vi "Format Fit Output.vi"(5 "Fit Model":T4, 7 "f(x,a)":T1, 8 "Error In":errorcluster, 9 "Fit Results":T2, 10 "Additional Data":variant, 11 "Data in":T3) -> (0 "Error Out":errorcluster, 1 "Fit Parameters Uncertainties Cluster":variant, 3 "Fit Parameters Cluster":variant)   [LabVIEW 2019]
uses:
  Fit Models.ctl
  <vilib>/gmath/NumericalOptimization/LM model function reference.ctl
  <vilib>/Utility/error.llb/DialogType.ctl
  Gaussian Fit Results v2.ctl
  Asymmetric Gaussian Fit Results v2.ctl
  Lorentzian Fit Results v2.ctl
  Asymmetric Lorentzian Fit Results v2.ctl
  Gaussian-Lorentzian Fit Results v2.ctl
  Lorentzian-Gaussian Fit Results v2.ctl
  D-Only Fixed Parameters.ctl
  Two H-Connected Gaussians Fit Parameters.ctl
  Two T-Connected Gaussians Fit Parameters.ctl
  Two H-Connected Asymmetric Gaussians Fit Parameters.ctl
  Two T-Connected Asymmetric Gaussians Fit Parameters.ctl
  Single Exponential Fit Parameters v2.ctl
  Double Exponential Fit Parameters v2.ctl
  2D Gaussian ACF Fit Results.ctl
  2D Gaussian + Blinking ACF Fit Results.ctl
  2D Gaussian + Flow ACF Fit Results.ctl
  3D Gaussian ACF Fit Results.ctl
  3D Gaussian + Blinking ACF Fit Results.ctl
  2D Gaussian ACF & 2D Gaussian ACF + Flow Fit Results.ctl
  <vilib>/Analysis/NI_AALPro.lvlib
  <vilib>/gmath/NI_Gmath.lvlib
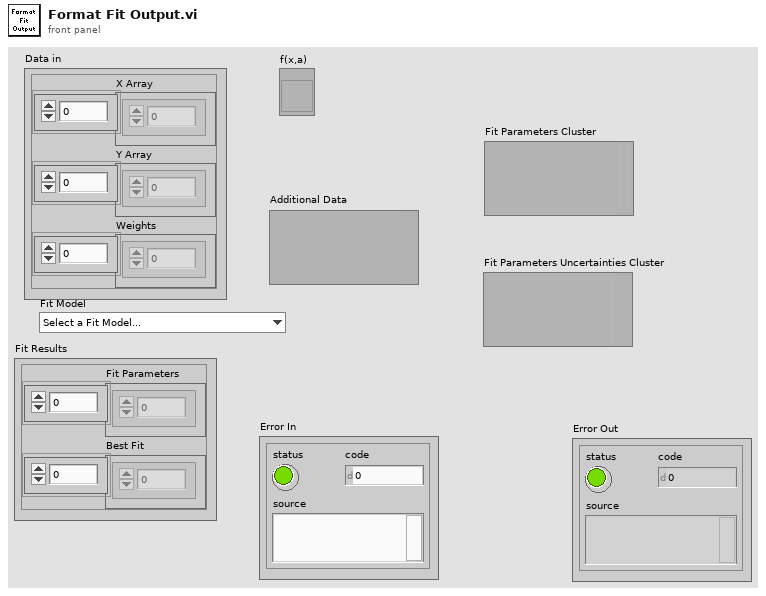
[diagram p1: front panel]
types:
  T1 = typedef "NI_Gmath.lvlib/LM model function reference.ctl" = refnum<vi>
  T2 = cluster{"Fit Parameters":dbl[], "Best Fit":dbl[]}
  T3 = cluster{"X Array":dbl[], "Y Array":dbl[], "Weights":dbl[]}
  T4 = typedef "Fit Models.ctl" = enum16{"Select a Fit Model...", "           Single Peak", "Gaussian", "Asymmetric Gaussian", "Lorentzian", "Asymmetric Lorentzian", "Gaussian/Lorentzian", "Lorentzian/Gaussian", "           Double Peak", "Two Gaussians", "Two Asymmetric Gaussians", "Two H-Connected Gaussians", "Two T-Connected Gaussians", "Two H-Connected Asymmetric Gaussians", "Two T-Connected Asymmetric Gaussians", "           Triple Peak", "Three Gaussians", "Three Asymmetric Gaussians", "              Decays", "Single Exponential", "Two Exponentials", "               ACF", "2D Gaussian ACF", "2D Gaussian + Blinking ACF", "2D Gaussian + Flow ACF", "3D Gaussian ACF", "3D Gaussian + Blinking ACF", "             Multiplot", "2D Gaussian ACF & 2D Gaussian + Flow ACF"}
  T5 = typedef "D-Only Fixed Parameters.ctl" = cluster{"Fix D-only Peak Location":bool, "Peak Location":dbl, "Fix D-only Peak FWHM":bool, "Peak FWHM":dbl}
  T6 = typedef "DialogType.ctl" = u16
  T7 = typedef "Gaussian Fit Results v2.ctl" = cluster{"Amplitude":dbl, "Peak":dbl, "SDV":dbl, "FWHM":dbl, "Integral":dbl, "RMSE":dbl, "R^2":dbl}
  T8 = typedef "Asymmetric Gaussian Fit Results v2.ctl" = cluster{"Amplitude":dbl, "Peak":dbl, "SDV-":dbl, "SDV+":dbl, "Mean":dbl, "SDV":dbl, "FWHM":dbl, "Integral":dbl, "RMSE":dbl, "R^2":dbl}
  T9 = typedef "Lorentzian Fit Results v2.ctl" = cluster{"Amplitude":dbl, "Peak":dbl, "FWHM":dbl, "Integral":dbl, "RMSE":dbl, "R^2":dbl}
  T10 = typedef "Asymmetric Lorentzian Fit Results v2.ctl" = cluster{"Amplitude":dbl, "Peak":dbl, "FWHM-":dbl, "FWHM+":dbl, "Integral":dbl, "RMSE":dbl, "R^2":dbl}
  T11 = typedef "Gaussian-Lorentzian Fit Results v2.ctl" = cluster{"Amplitude":dbl, "Peak":dbl, "SDV-":dbl, "FWHM+":dbl, "Mean":dbl, "FWHM":dbl, "Integral":dbl, " RMSE":dbl, "R^2":dbl}
  T12 = typedef "Lorentzian-Gaussian Fit Results v2.ctl" = cluster{"Amplitude":dbl, "Peak":dbl, "FWHM-":dbl, "SDV+":dbl, "Mean":dbl, "FWHM":dbl, "Integral":dbl, "RMSE":dbl, "R^2":dbl}
  T13 = typedef "Two H-Connected Gaussians Fit Parameters.ctl" = cluster{"Gaussian Parameters":T7[], "Bridge Amplitude ":dbl}
  T14 = typedef "Two T-Connected Gaussians Fit Parameters.ctl" = cluster{"Gaussian Parameters":T7[], "Bridge Amplitude ":dbl, "Bridge Slope":dbl}
  T15 = typedef "Two H-Connected Asymmetric Gaussians Fit Parameters.ctl" = cluster{"Asymmetric Gaussian Parameters":T8[], "Bridge Amplitude":dbl}
  T16 = typedef "Two T-Connected Asymmetric Gaussians Fit Parameters.ctl" = cluster{"Asymmetric Gaussian Parameters":T8[], "Bridge Amplitude":dbl, "Bridge Slope":dbl}
  T17 = typedef "Single Exponential Fit Parameters v2.ctl" = cluster{"Amplitude":dbl, "Time Constant":dbl, "Mean":dbl, "SDV":dbl, "FWHM":dbl, "Integral":dbl, "MSE":dbl, "R^2":dbl}
  T18 = typedef "Double Exponential Fit Parameters v2.ctl" = cluster{"A1":dbl, "tau1":dbl, "A2":dbl, "tau2":dbl, "Mean":dbl, "SDV":dbl, "Integral":dbl, "MSE":dbl, "R^2":dbl}
  T19 = typedef "2D Gaussian ACF Fit Results.ctl" = cluster{"Amplitude":dbl, "Diffusion Time":dbl, "RMSE":dbl, "R^2":dbl}
  T20 = typedef "2D Gaussian + Blinking ACF Fit Results.ctl" = cluster{"Amplitude":dbl, "Diffusion Time":dbl, "Blinking Fraction":dbl, "Blinking Time Constant":dbl, "RMSE":dbl, "R^2":dbl}
  T21 = typedef "2D Gaussian + Flow ACF Fit Results.ctl" = cluster{"Amplitude":dbl, "Diffusion Time":dbl, "Translation Time":dbl, "RMSE":dbl, "R^2":dbl}
  T22 = typedef "3D Gaussian ACF Fit Results.ctl" = cluster{"Amplitude":dbl, "Diffusion Time":dbl, "Aspect Ratio":dbl, "RMSE":dbl, "R^2":dbl}
  T23 = typedef "3D Gaussian + Blinking ACF Fit Results.ctl" = cluster{"Amplitude":dbl, "Diffusion Time":dbl, "Aspect Ratio":dbl, "Blinking Fraction":dbl, "Blinking Time Constant":dbl, "RMSE":dbl, "R^2":dbl}
  T24 = typedef "2D Gaussian ACF & 2D Gaussian ACF + Flow Fit Results.ctl" = cluster{"Amplitude 1":dbl, "Diffusion Time":dbl, "Amplitude 2":dbl, "Translation Time":dbl, "RMSE":dbl, "R^2":dbl}
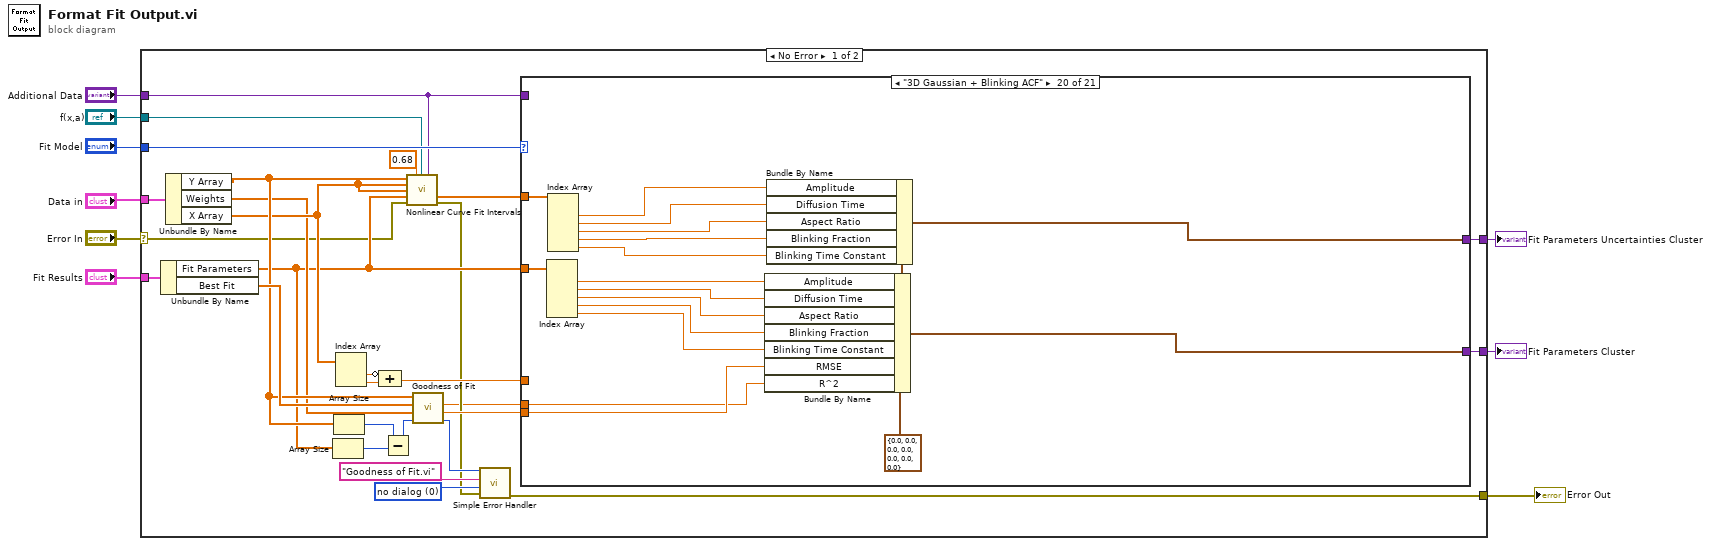
[diagram p0: block diagram]
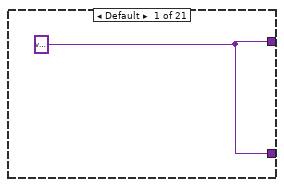
[diagram p2: hidden frame]
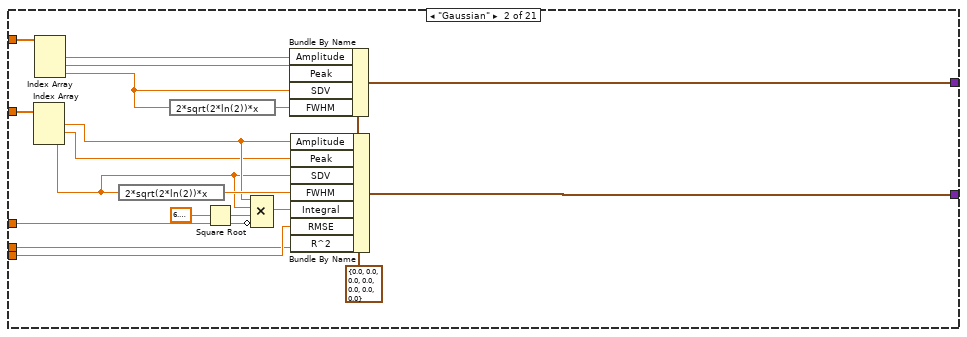
[diagram p3: hidden frame]
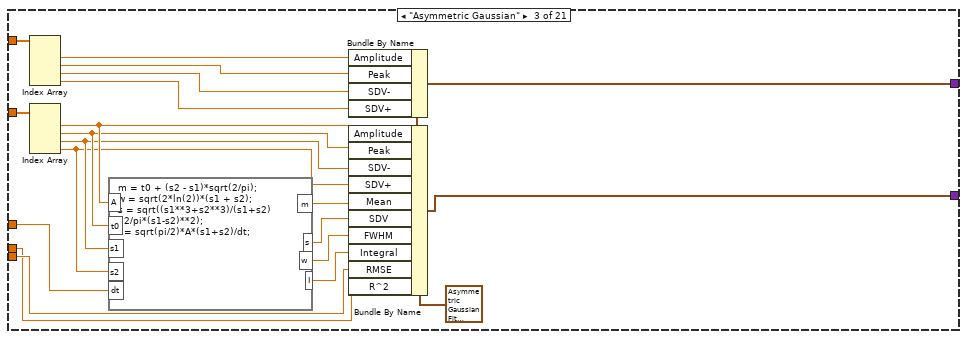
[diagram p4: hidden frame]
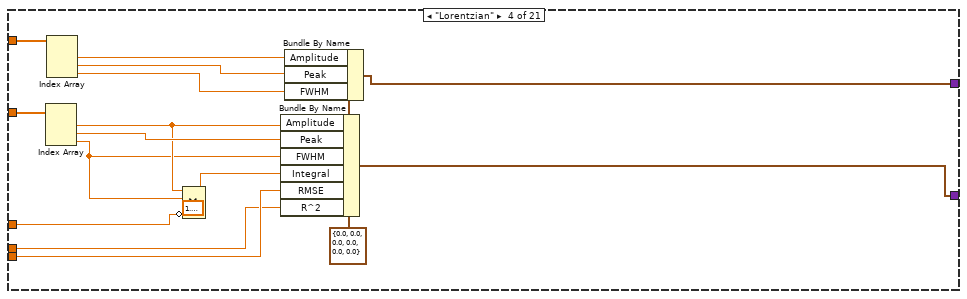
[diagram p5: hidden frame]
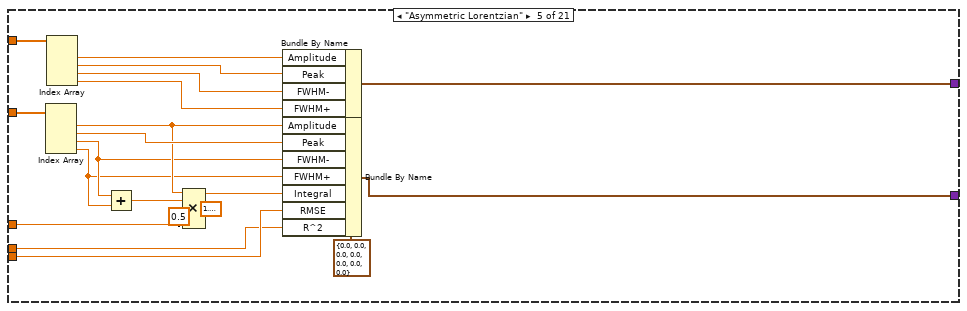
[diagram p6: hidden frame]
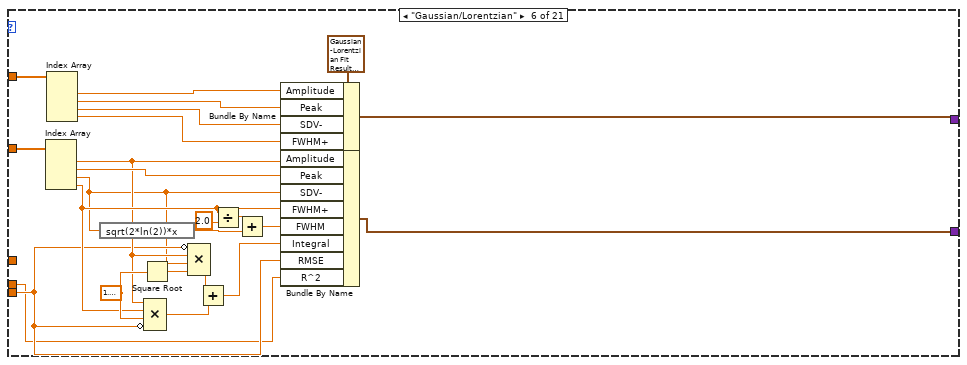
[diagram p7: hidden frame]
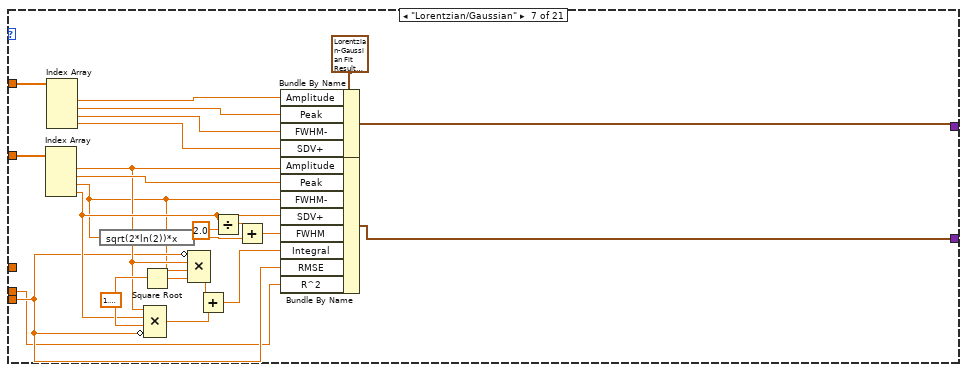
[diagram p8: hidden frame]
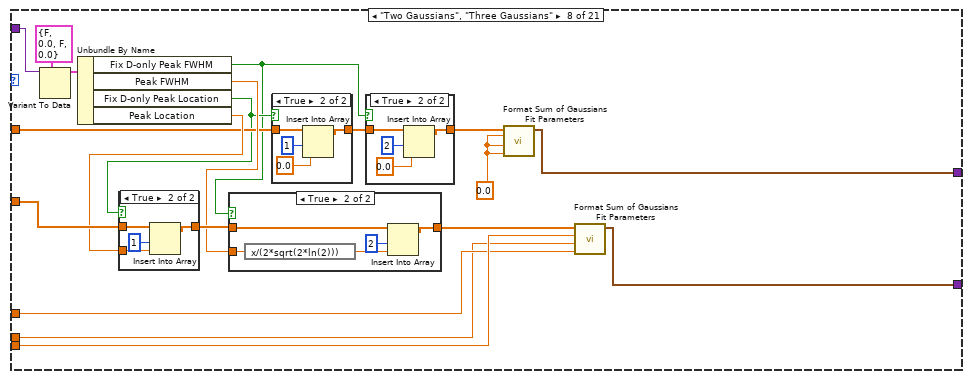
[diagram p9: hidden frame]
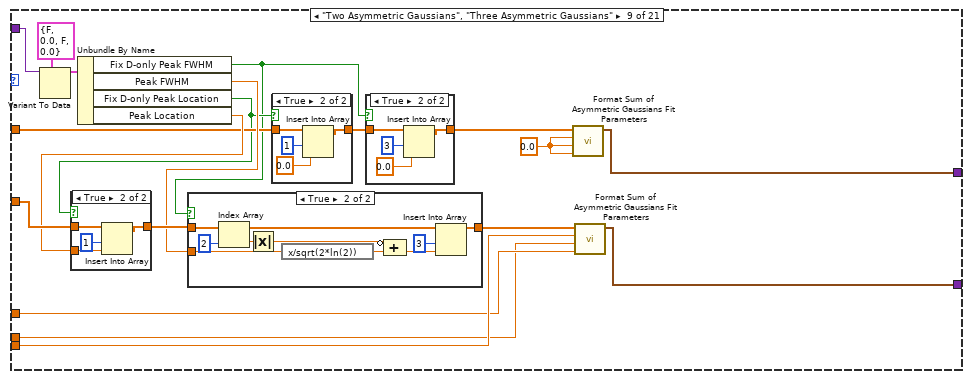
[diagram p14: hidden frame]
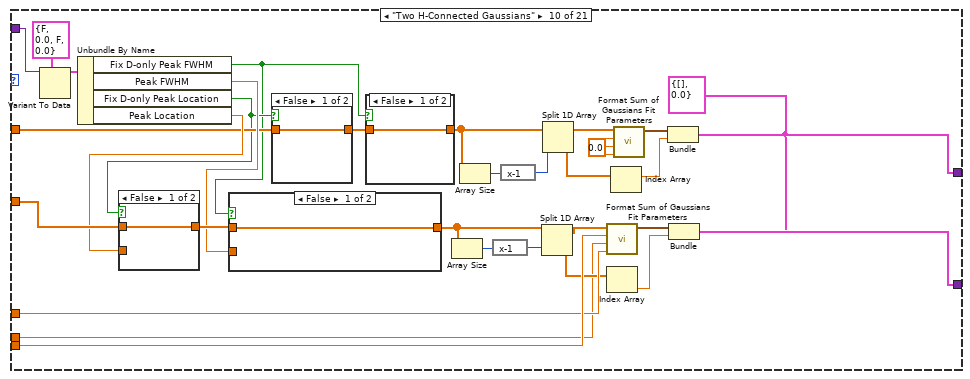
[diagram p19: hidden frame]
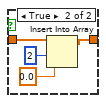
[diagram p20: hidden frame]
diagram:
  n1 = case shown="No Error" "Error In" {
    selector: "Error In" -> [w19 w589]
    tunnel: [w37 _] -> w9
    tunnel: [w36 _] -> w8
    tunnel: "Data in" -> [w28 _]
    tunnel: "Fit Results" -> [w27 _]
    tunnel: "Fit Model" -> [w25 _]
    tunnel: "f(x,a)" -> [w18 _]
    tunnel: [w13 w589] -> w2
    tunnel: "Additional Data" -> [w11 _]
    frame No Error {
      w15 = T6 0 items=["no dialog", "OK message", "continue or stop message", "OK message + warnings", "continue/stop + warnings"] ("type of dialog (OK msg:1)")
      n2 = Unbundle By Name(w27) -> ("Fit Parameters"=w21:dbl[], "Best Fit"=w26:dbl[])
      n3 = Unbundle By Name(w28) -> ("Y Array"=w24:dbl[], "Weights"=w22:dbl[], "X Array"=w23:dbl[])
      n4 = Array Size(array=w21) -> (size(s)=w31:i32)
      n5 = Array Size(array=w24) -> (size(s)=w32:i32)
      n6 = Index Array(array=w23) -> (element #1=w33:dbl, element #2=w35:dbl)  [unwired: 2 in]
      n7 = Compound Arithmetic op=ADD(invert w33, w35) -> (w34:dbl)
      n8 = Subtract(x=w32, y=w31) -> (x-y=w30:i32)
      n9 = call <vilib>:"Nonlinear Curve Fit Intervals.vi"("Y"=w24, "confidence level"=0.68, "f(x,a)"=w18, "data"=w11, "X"=w23, "Weight"=w23, "best fit parameters"=w21, "error in (no error)"=w19) -> ("delta best fit parameters"=w20:dbl[], "error out"=w14:errorcluster)  [unwired: 4 in, 2 out]
      n10 = call <vilib>:"Goodness of Fit.vi"("degree of freedom"=w30, "Weight"=w22, "Best Fit"=w26, "Y"=w24) -> ("error"=w17:i32, "RMSE"=w29:dbl, "R-square"=w10:dbl)  [unwired: 4 in, 1 out]
      n11 = call <vilib>:"Simple Error Handler.vi"("error code (no error:0)"=w17, "error source (\" \")"="Goodness of Fit.vi" ("error source (\" \")"), "type of dialog (OK msg:1)"=w15, "error in (no error)"=w14) -> ("error out"=w13:errorcluster)  [unwired: 1 in, 4 out]
      n12 = case shown="\"3D Gaussian + Blinking ACF\"" w25 {
        tunnel: [w38 w45 w71 w79 w103 w131 w155 w165 w205 w263 w318 w371 w430 w472 w498 w511 w526 w539 w554 w571 w586] -> w37
        tunnel: [w38 w44 w70 w91 w102 w130 w154 w164 w204 w264 w319 w372 w431 w471 w490 w510 w525 w538 w553 w570 w585] -> w36
        tunnel: w34 -> [_ w48 w60 w86 w108 _ _ w167 w207 w265 w320 w373 w432 w475 w496 _ _ _ _ _ _]
        tunnel: w29 -> [_ w47 w69 w92 w112 w116 w141 w168 w208 w266 w321 w374 w433 w476 w492 w513 w528 w541 w556 w573 w588]
        tunnel: w21 -> [_ w46 w77 w93 w113 w137 w161 w177 w217 w274 w329 w382 w441 w480 w497 w512 w527 w540 w555 w572 w587]
        tunnel: w20 -> [_ w43 w76 w84 w107 w135 w159 w173 w213 w270 w325 w378 w437 w483 w503 w509 w524 w537 w552 w569 w584]
        tunnel: w11 -> [_ _ _ _ _ _ _ w179 w219 w276 w331 w384 w443 _ _ _ _ _ _ _ _]
        tunnel: w10 -> [_ w39 w58 w78 w94 w114 w138 w163 w202 w247 w299 w354 w412 w470 w485 w507 w522 w535 w551 w567 w582]
        frame Default {
          w38 = variant
        }
        frame "Gaussian" {
          w56 = T7 {"Amplitude"=0.0, "Peak"=0.0, "SDV"=0.0, "FWHM"=0.0, "Integral"=0.0, "RMSE"=0.0, "R^2"=0.0} ("Gaussian Fit Parameters")
          n13 = Index Array(array=w46) -> (element #1=w51:dbl, element #2=w50:dbl, element #3=w49:dbl)  [unwired: 3 in]
          n14 = Index Array(array=w43) -> (element #1=w42:dbl, element #2=w41:dbl, element #3=w40:dbl)  [unwired: 3 in]
          n15 = expression code="2*sqrt(2*ln(2))*x"(w49) -> (w55:dbl)
          n16 = expression code="2*sqrt(2*ln(2))*x"(w40) -> (w57:dbl)
          n17 = Square Root(x=6.283185307179586) -> (sqrt(x)=w53:dbl)
          n18 = Compound Arithmetic op=MULTIPLY(w51, w49, w53, invert w48) -> (w54:dbl)
          n19 = Bundle By Name(cluster=w56, "Amplitude"=w42, "Peak"=w41, "SDV"=w40, "FWHM"=w57) -> (w45:T7)
          n20 = Bundle By Name(cluster=w56, "Amplitude"=w51, "Peak"=w50, "SDV"=w49, "FWHM"=w55, "Integral"=w54, "RMSE"=w47, "R^2"=w39) -> (w44:T7)
        }
        frame "Asymmetric Gaussian" {
          w75 = T8 {"Amplitude"=0.0, "Peak"=0.0, "SDV-"=0.0, "SDV+"=0.0, "Mean"=0.0, "SDV"=0.0, "FWHM"=0.0, "Integral"=0.0, "RMSE"=0.0, "R^2"=0.0} ("Lorentz Fit Parameters")
          n21 = Index Array(array=w76) -> (element #1=w74:dbl, element #2=w73:dbl, element #3=w72:dbl, element #4=w59:dbl)  [unwired: 4 in]
          n22 = Index Array(array=w77) -> (element #1=w64:dbl, element #2=w63:dbl, element #3=w62:dbl, element #4=w61:dbl)  [unwired: 4 in]
          n23 = formula code="m = t0 + (s2 - s1)*sqrt(2/pi);\nw = sqrt(2*ln(2))*(s1 + s2);\ns = sqrt((s1**3+s2**3)/(s1+s2)\n- 2/pi*(s1-s2)**2);\nI = sqrt(pi/2)*A*(s1+s2)/dt;"("t0"=w63, "s1"=w62, "s2"=w61, "A"=w64, "dt"=w60) -> ("m"=w65:dbl, "w"=w67:dbl, "s"=w66:dbl, "I"=w68:dbl)
          n24 = Bundle By Name(cluster=w75, "Amplitude"=w74, "Peak"=w73, "SDV-"=w72, "SDV+"=w59) -> (w71:T8)
          n25 = Bundle By Name(cluster=w75, "Amplitude"=w64, "Peak"=w63, "SDV-"=w62, "SDV+"=w61, "Mean"=w65, "SDV"=w66, "FWHM"=w67, "Integral"=w68, "RMSE"=w69, "R^2"=w58) -> (w70:T8)
        }
        frame "Lorentzian" {
          w83 = T9 {"Amplitude"=0.0, "Peak"=0.0, "FWHM"=0.0, "Integral"=0.0, "RMSE"=0.0, "R^2"=0.0} ("Lorentz Fit Parameters")
          n26 = Index Array(array=w93) -> (element #1=w89:dbl, element #2=w90:dbl, element #3=w88:dbl)  [unwired: 3 in]
          n27 = Index Array(array=w84) -> (element #1=w82:dbl, element #2=w81:dbl, element #3=w80:dbl)  [unwired: 3 in]
          n28 = Compound Arithmetic op=MULTIPLY(w89, w88, 1.5707963267948966, invert w86) -> (w85:dbl)
          n29 = Bundle By Name(cluster=w83, "Amplitude"=w89, "Peak"=w90, "FWHM"=w88, "Integral"=w85, "RMSE"=w92, "R^2"=w78) -> (w91:T9)
          n30 = Bundle By Name(cluster=w83, "Amplitude"=w82, "Peak"=w81, "FWHM"=w80) -> (w79:T9)
        }
        frame "Asymmetric Lorentzian" {
          w101 = T10 {"Amplitude"=0.0, "Peak"=0.0, "FWHM-"=0.0, "FWHM+"=0.0, "Integral"=0.0, "RMSE"=0.0, "R^2"=0.0} ("Asymmetric Lorentz Fit Parameters")
          n31 = Index Array(array=w113) -> (element #1=w110:dbl, element #2=w111:dbl, element #3=w99:dbl, element #4=w98:dbl)  [unwired: 4 in]
          n32 = Index Array(array=w107) -> (element #1=w106:dbl, element #2=w105:dbl, element #3=w104:dbl, element #4=w100:dbl)  [unwired: 4 in]
          n33 = Add(x=w99, y=w98) -> (x+y=w97:dbl)
          n34 = Compound Arithmetic op=MULTIPLY(w110, w97, 1.5707963267948966, 0.5 ("value"), invert w108) -> (w95:dbl)
          n35 = Bundle By Name(cluster=w101, "Amplitude"=w106, "Peak"=w105, "FWHM-"=w104, "FWHM+"=w100) -> (w103:T10)
          n36 = Bundle By Name(cluster=w101, "Amplitude"=w110, "Peak"=w111, "FWHM-"=w99, "FWHM+"=w98, "Integral"=w95, "RMSE"=w112, "R^2"=w94) -> (w102:T10)
        }
        frame "Gaussian/Lorentzian" {
          w126 = 1.5707963267948966
          w129 = T11 {"Amplitude"=0.0, "Peak"=0.0, "SDV-"=0.0, "FWHM+"=0.0, "Mean"=0.0, "FWHM"=0.0, "Integral"=0.0, " RMSE"=0.0, "R^2"=0.0} ("Gaussian/Lorentzian Fit Parameters")
          n37 = Index Array(array=w137) -> (element #1=w117:dbl, element #2=w136:dbl, element #3=w115:dbl, element #4=w118:dbl)  [unwired: 4 in]
          n38 = Index Array(array=w135) -> (element #1=w134:dbl, element #2=w133:dbl, element #3=w132:dbl, element #4=w128:dbl)  [unwired: 4 in]
          n39 = expression code="sqrt(2*ln(2))*x"(w115) -> (w121:dbl)
          n40 = Square Root(x=w126) -> (sqrt(x)=w127:dbl)
          n41 = Compound Arithmetic op=MULTIPLY(w117, w118, w126, invert w116) -> (w125:dbl)
          n42 = Compound Arithmetic op=MULTIPLY(invert w116, w117, w115, w127) -> (w124:dbl)
          n43 = Add(x=w124, y=w125) -> (x+y=w119:dbl)
          n44 = Divide(x=w118, y=2.0) -> (x/y=w123:dbl)
          n45 = Add(x=w123, y=w121) -> (x+y=w120:dbl)
          n46 = Bundle By Name(cluster=w129, "Amplitude"=w134, "Peak"=w133, "SDV-"=w132, "FWHM+"=w128) -> (w131:T11)
          n47 = Bundle By Name(cluster=w129, "Amplitude"=w117, "Peak"=w136, "SDV-"=w115, "FWHM+"=w118, "FWHM"=w120, "Integral"=w119, "RMSE"=w116, "R^2"=w114) -> (w130:T11)
        }
        frame "Lorentzian/Gaussian" {
          w139 = T12 {"Amplitude"=0.0, "Peak"=0.0, "FWHM-"=0.0, "SDV+"=0.0, "Mean"=0.0, "FWHM"=0.0, "Integral"=0.0, "RMSE"=0.0, "R^2"=0.0} ("Lorentzian/Gaussian Fit Parameters")
          w151 = 1.5707963267948966
          n48 = Index Array(array=w161) -> (element #1=w142:dbl, element #2=w160:dbl, element #3=w140:dbl, element #4=w143:dbl)  [unwired: 4 in]
          n49 = Index Array(array=w159) -> (element #1=w158:dbl, element #2=w157:dbl, element #3=w156:dbl, element #4=w153:dbl)  [unwired: 4 in]
          n50 = expression code="sqrt(2*ln(2))*x"(w140) -> (w146:dbl)
          n51 = Square Root(x=w151) -> (sqrt(x)=w152:dbl)
          n52 = Compound Arithmetic op=MULTIPLY(w142, w143, w151, invert w141) -> (w150:dbl)
          n53 = Compound Arithmetic op=MULTIPLY(invert w141, w142, w140, w152) -> (w149:dbl)
          n54 = Add(x=w149, y=w150) -> (x+y=w144:dbl)
          n55 = Divide(x=w143, y=2.0) -> (x/y=w148:dbl)
          n56 = Add(x=w148, y=w146) -> (x+y=w145:dbl)
          n57 = Bundle By Name(cluster=w139, "Amplitude"=w158, "Peak"=w157, "FWHM-"=w156, "SDV+"=w153) -> (w155:T12)
          n58 = Bundle By Name(cluster=w139, "Amplitude"=w142, "Peak"=w160, "FWHM-"=w140, "SDV+"=w143, "FWHM"=w145, "Integral"=w144, "RMSE"=w141, "R^2"=w138) -> (w154:T12)
        }
        frame "Two Gaussians", "Three Gaussians" {
          w162 = 0.0 ("MSE")
          n59 = Variant To Data(type=T5 {"Fix D-only Peak Location"=FALSE, "Peak Location"=0.0, "Fix D-only Peak FWHM"=FALSE, "Peak FWHM"=0.0} ("Fixed Parameters"), Variant=w179) -> (data=w178:T5)  [unwired: 1 in, 1 out]
          n60 = Unbundle By Name(w178) -> ("Fix D-only Peak FWHM"=w170:bool, "Peak FWHM"=w174:dbl, "Fix D-only Peak Location"=w172:bool, "Peak Location"=w175:dbl)
          n61 = case shown="True" w172 {
            tunnel: w177 -> [w197 w201]
            tunnel: [w197 w200] -> w176
            tunnel: w175 -> [_ w198]
            frame False {
            }
            frame True {
              n62 = Insert Into Array(array=w201, index=1 ("length"), new element=w198) -> (w200:dbl[])
            }
          }
          n63 = case shown="True" w170 {
            tunnel: w176 -> [w191 w196]
            tunnel: [w191 w195] -> w169
            tunnel: w174 -> [_ w193]
            frame False {
            }
            frame True {
              n64 = expression code="x/(2*sqrt(2*ln(2)))"(w193) -> (w192:dbl)
              n65 = Insert Into Array(array=w196, index=2, new element=w192) -> (w195:dbl[])
            }
          }
          n66 = case shown="True" w172 {
            tunnel: w173 -> [w186 w190]
            tunnel: [w186 w189] -> w171
            frame False {
            }
            frame True {
              n67 = Insert Into Array(array=w190, index=1 ("length"), new element=0.0 ("new element/subarray")) -> (w189:dbl[])
            }
          }
          n68 = case shown="True" w170 {
            tunnel: w171 -> [w181 w185]
            tunnel: [w181 w184] -> w166
            frame False {
            }
            frame True {
              n69 = Insert Into Array(array=w185, index=2, new element=0.0 ("new element/subarray")) -> (w184:dbl[])
            }
          }
          n70 = call "Format Sum of Gaussians Fit Parameters.vi"("Step Size"=w162, "R^2"=w162, "MSE"=w162, "Best Fit Parameters"=w166) -> ("Array of Gaussian Fit Parameters"=w165:T7[])  [unwired: 6 in, 1 out]
          n71 = call "Format Sum of Gaussians Fit Parameters.vi"("Step Size"=w167, "R^2"=w163, "MSE"=w168, "Best Fit Parameters"=w169) -> ("Array of Gaussian Fit Parameters"=w164:T7[])  [unwired: 6 in, 1 out]
        }
        frame "Two Asymmetric Gaussians", "Three Asymmetric Gaussians" {
          w203 = 0.0 ("MSE")
          n72 = Variant To Data(type=T5 {"Fix D-only Peak Location"=FALSE, "Peak Location"=0.0, "Fix D-only Peak FWHM"=FALSE, "Peak FWHM"=0.0} ("Fixed Parameters"), Variant=w219) -> (data=w218:T5)  [unwired: 1 in, 1 out]
          n73 = Unbundle By Name(w218) -> ("Fix D-only Peak FWHM"=w210:bool, "Peak FWHM"=w214:dbl, "Fix D-only Peak Location"=w212:bool, "Peak Location"=w215:dbl)
          n74 = case shown="True" w212 {
            tunnel: w217 -> [w241 w245]
            tunnel: [w241 w244] -> w216
            tunnel: w215 -> [_ w242]
            frame False {
            }
            frame True {
              n75 = Insert Into Array(array=w245, index=1 ("length"), new element=w242) -> (w244:dbl[])
            }
          }
          n76 = case shown="True" w210 {
            tunnel: w216 -> [w231 w236]
            tunnel: [w231 w240] -> w209
            tunnel: w214 -> [_ w238]
            frame False {
            }
            frame True {
              n77 = Index Array(array=w236, index=2) -> (element=w233:dbl)
              n78 = Absolute Value(x=w233) -> (abs(x)=w232:dbl)
              n79 = expression code="x/sqrt(2*ln(2))"(w238) -> (w237:dbl)
              n80 = Compound Arithmetic op=ADD(invert w232, w237) -> (w234:dbl)
              n81 = Insert Into Array(array=w236, index=3, new element=w234) -> (w240:dbl[])
            }
          }
          n82 = case shown="True" w212 {
            tunnel: w213 -> [w226 w230]
            tunnel: [w226 w229] -> w211
            frame False {
            }
            frame True {
              n83 = Insert Into Array(array=w230, index=1 ("length"), new element=0.0 ("new element/subarray")) -> (w229:dbl[])
            }
          }
          n84 = case shown="True" w210 {
            tunnel: w211 -> [w221 w225]
            tunnel: [w221 w224] -> w206
            frame False {
            }
            frame True {
              n85 = Insert Into Array(array=w225, index=3, new element=0.0 ("new element/subarray")) -> (w224:dbl[])
            }
          }
          n86 = call "Format Sum of Asymmetric Gaussians Fit Parameters.vi"("Step Size"=w203, "R^2"=w203, "MSE"=w203, "Best Fit Parameters"=w206) -> ("Array of Asymmetric Gaussian Fit Parameters"=w205:T8[])  [unwired: 6 in, 1 out]
          n87 = call "Format Sum of Asymmetric Gaussians Fit Parameters.vi"("Step Size"=w207, "R^2"=w202, "MSE"=w208, "Best Fit Parameters"=w209) -> ("Array of Asymmetric Gaussian Fit Parameters"=w204:T8[])  [unwired: 6 in, 1 out]
        }
        frame "Two H-Connected Gaussians" {
          w250 = T13 {"Gaussian Parameters"=[], "Bridge Amplitude "=0.0} ("Bridged Gaussians Parameters")
          w246 = 0.0 ("MSE")
          n88 = Variant To Data(type=T5 {"Fix D-only Peak Location"=FALSE, "Peak Location"=0.0, "Fix D-only Peak FWHM"=FALSE, "Peak FWHM"=0.0} ("Fixed Parameters"), Variant=w276) -> (data=w275:T5)  [unwired: 1 in, 1 out]
          n89 = Unbundle By Name(w275) -> ("Fix D-only Peak FWHM"=w267:bool, "Peak FWHM"=w271:dbl, "Fix D-only Peak Location"=w269:bool, "Peak Location"=w272:dbl)
          n90 = case shown="False" w269 {
            tunnel: w274 -> [w294 w298]
            tunnel: [w294 w297] -> w273
            tunnel: w272 -> [_ w295]
            frame False {
            }
            frame True {
              n91 = Insert Into Array(array=w298, index=1 ("length"), new element=w295) -> (w297:dbl[])
            }
          }
          n92 = case shown="False" w267 {
            tunnel: w273 -> [w288 w293]
            tunnel: [w288 w292] -> w257
            tunnel: w271 -> [_ w290]
            frame False {
            }
            frame True {
              n93 = expression code="x/(2*sqrt(2*ln(2)))"(w290) -> (w289:dbl)
              n94 = Insert Into Array(array=w293, index=2, new element=w289) -> (w292:dbl[])
            }
          }
          n95 = case shown="False" w269 {
            tunnel: w270 -> [w283 w287]
            tunnel: [w283 w286] -> w268
            frame False {
            }
            frame True {
              n96 = Insert Into Array(array=w287, index=1 ("length"), new element=0.0 ("new element/subarray")) -> (w286:dbl[])
            }
          }
          n97 = case shown="False" w267 {
            tunnel: w268 -> [w278 w282]
            tunnel: [w278 w281] -> w261
            frame False {
            }
            frame True {
              n98 = Insert Into Array(array=w282, index=2, new element=0.0 ("new element/subarray")) -> (w281:dbl[])
            }
          }
          n99 = Array Size(array=w257) -> (size(s)=w258:i32)
          n100 = Array Size(array=w261) -> (size(s)=w260:i32)
          n101 = expression code="x-1"(w258) -> (w256:i32)
          n102 = expression code="x-1"(w260) -> (w259:i32)
          n103 = Split 1D Array(array=w257, index=w256) -> (first subarray=w255:dbl[], second subarray=w249:dbl[])
          n104 = Split 1D Array(array=w261, index=w259) -> (first subarray=w262:dbl[], second subarray=w253:dbl[])
          n105 = call "Format Sum of Gaussians Fit Parameters.vi"("Step Size"=w265, "R^2"=w247, "MSE"=w266, "Best Fit Parameters"=w255) -> ("Array of Gaussian Fit Parameters"=w251:T7[])  [unwired: 6 in, 1 out]
          n106 = Index Array(array=w249) -> (element=w248:dbl)  [unwired: 1 in]
          n107 = Index Array(array=w253) -> (element=w252:dbl)  [unwired: 1 in]
          n108 = call "Format Sum of Gaussians Fit Parameters.vi"("Step Size"=w246, "R^2"=w246, "MSE"=w246, "Best Fit Parameters"=w262) -> ("Array of Gaussian Fit Parameters"=w254:T7[])  [unwired: 6 in, 1 out]
          n109 = Bundle(cluster=w250, "Gaussian Parameters"=w254, "Bridge Amplitude"=w252) -> (w263:T13)
          n110 = Bundle(cluster=w250, "Gaussian Parameters"=w251, "Bridge Amplitude"=w248) -> (w264:T13)
        }
        frame "Two T-Connected Gaussians" {
          w305 = T14 {"Gaussian Parameters"=[], "Bridge Amplitude "=0.0, "Bridge Slope"=0.0} ("Bridged Gaussians Parameters")
          w300 = 0.0 ("MSE")
          n111 = Variant To Data(type=T5 {"Fix D-only Peak Location"=FALSE, "Peak Location"=0.0, "Fix D-only Peak FWHM"=FALSE, "Peak FWHM"=0.0} ("Fixed Parameters"), Variant=w331) -> (data=w330:T5)  [unwired: 1 in, 1 out]
          n112 = Unbundle By Name(w330) -> ("Fix D-only Peak FWHM"=w322:bool, "Peak FWHM"=w326:dbl, "Fix D-only Peak Location"=w324:bool, "Peak Location"=w327:dbl)
          n113 = case shown="True" w324 {
            tunnel: w329 -> [w349 w353]
            tunnel: [w349 w352] -> w328
            tunnel: w327 -> [_ w350]
            frame False {
            }
            frame True {
              n114 = Insert Into Array(array=w353, index=1 ("length"), new element=w350) -> (w352:dbl[])
            }
          }
          n115 = case shown="True" w322 {
            tunnel: w328 -> [w343 w348]
            tunnel: [w343 w347] -> w312
            tunnel: w326 -> [_ w345]
            frame False {
            }
            frame True {
              n116 = expression code="x/(2*sqrt(2*ln(2)))"(w345) -> (w344:dbl)
              n117 = Insert Into Array(array=w348, index=2, new element=w344) -> (w347:dbl[])
            }
          }
          n118 = case shown="True" w324 {
            tunnel: w325 -> [w338 w342]
            tunnel: [w338 w341] -> w323
            frame False {
            }
            frame True {
              n119 = Insert Into Array(array=w342, index=1 ("length"), new element=0.0 ("new element/subarray")) -> (w341:dbl[])
            }
          }
          n120 = case shown="True" w322 {
            tunnel: w323 -> [w333 w337]
            tunnel: [w333 w336] -> w316
            frame False {
            }
            frame True {
              n121 = Insert Into Array(array=w337, index=2, new element=0.0 ("new element/subarray")) -> (w336:dbl[])
            }
          }
          n122 = Array Size(array=w312) -> (size(s)=w313:i32)
          n123 = Array Size(array=w316) -> (size(s)=w315:i32)
          n124 = expression code="x-2"(w313) -> (w311:i32)
          n125 = expression code="x-2"(w315) -> (w314:i32)
          n126 = Split 1D Array(array=w312, index=w311) -> (first subarray=w310:dbl[], second subarray=w304:dbl[])
          n127 = Split 1D Array(array=w316, index=w314) -> (first subarray=w317:dbl[], second subarray=w308:dbl[])
          n128 = call "Format Sum of Gaussians Fit Parameters.vi"("Step Size"=w320, "R^2"=w299, "MSE"=w321, "Best Fit Parameters"=w310) -> ("Array of Gaussian Fit Parameters"=w306:T7[])  [unwired: 6 in, 1 out]
          n129 = Index Array(array=w304) -> (element #1=w303:dbl, element #2=w301:dbl)  [unwired: 2 in]
          n130 = Index Array(array=w308) -> (element #1=w307:dbl, element #2=w302:dbl)  [unwired: 2 in]
          n131 = call "Format Sum of Gaussians Fit Parameters.vi"("Step Size"=w300, "R^2"=w300, "MSE"=w300, "Best Fit Parameters"=w317) -> ("Array of Gaussian Fit Parameters"=w309:T7[])  [unwired: 6 in, 1 out]
          n132 = Bundle By Name(cluster=w305, "Gaussian Parameters"=w309, "Bridge Amplitude"=w307, "Bridge Slope"=w302) -> (w318:T14)
          n133 = Bundle By Name(cluster=w305, "Gaussian Parameters"=w306, "Bridge Amplitude"=w303, "Bridge Slope"=w301) -> (w319:T14)
        }
        frame "Two H-Connected Asymmetric Gaussians" {
          w362 = T15 {"Asymmetric Gaussian Parameters"=[], "Bridge Amplitude"=0.0} ("output cluster")
          w355 = 0.0 ("MSE")
          n134 = Variant To Data(type=T5 {"Fix D-only Peak Location"=FALSE, "Peak Location"=0.0, "Fix D-only Peak FWHM"=FALSE, "Peak FWHM"=0.0} ("Fixed Parameters"), Variant=w384) -> (data=w383:T5)  [unwired: 1 in, 1 out]
          n135 = Unbundle By Name(w383) -> ("Fix D-only Peak FWHM"=w375:bool, "Peak FWHM"=w379:dbl, "Fix D-only Peak Location"=w377:bool, "Peak Location"=w380:dbl)
          n136 = case shown="True" w377 {
            tunnel: w382 -> [w406 w410]
            tunnel: [w406 w409] -> w381
            tunnel: w380 -> [_ w407]
            frame False {
            }
            frame True {
              n137 = Insert Into Array(array=w410, index=1 ("length"), new element=w407) -> (w409:dbl[])
            }
          }
          n138 = case shown="True" w375 {
            tunnel: w381 -> [w396 w401]
            tunnel: [w396 w405] -> w358
            tunnel: w379 -> [_ w403]
            frame False {
            }
            frame True {
              n139 = Index Array(array=w401, index=2) -> (element=w398:dbl)
              n140 = Absolute Value(x=w398) -> (abs(x)=w397:dbl)
              n141 = expression code="x/sqrt(2*ln(2))"(w403) -> (w402:dbl)
              n142 = Compound Arithmetic op=ADD(invert w397, w402) -> (w399:dbl)
              n143 = Insert Into Array(array=w401, index=3, new element=w399) -> (w405:dbl[])
            }
          }
          n144 = case shown="True" w377 {
            tunnel: w378 -> [w391 w395]
            tunnel: [w391 w394] -> w376
            frame False {
            }
            frame True {
              n145 = Insert Into Array(array=w395, index=1 ("length"), new element=0.0 ("new element/subarray")) -> (w394:dbl[])
            }
          }
          n146 = case shown="True" w375 {
            tunnel: w376 -> [w386 w390]
            tunnel: [w386 w389] -> w368
            frame False {
            }
            frame True {
              n147 = Insert Into Array(array=w390, index=3, new element=0.0 ("new element/subarray")) -> (w389:dbl[])
            }
          }
          n148 = Array Size(array=w368) -> (size(s)=w370:i32)
          n149 = Array Size(array=w358) -> (size(s)=w360:i32)
          n150 = expression code="x-1"(w370) -> (w369:i32)
          n151 = expression code="x-1"(w360) -> (w361:i32)
          n152 = Split 1D Array(array=w368, index=w369) -> (first subarray=w367:dbl[], second subarray=w365:dbl[])
          n153 = Split 1D Array(array=w358, index=w361) -> (first subarray=w359:dbl[], second subarray=w357:dbl[])
          n154 = call "Format Sum of Asymmetric Gaussians Fit Parameters.vi"("Step Size"=w355, "R^2"=w355, "MSE"=w355, "Best Fit Parameters"=w367) -> ("Array of Asymmetric Gaussian Fit Parameters"=w366:T8[])  [unwired: 6 in, 1 out]
          n155 = Index Array(array=w365) -> (element=w364:dbl)  [unwired: 1 in]
          n156 = call "Format Sum of Asymmetric Gaussians Fit Parameters.vi"("Step Size"=w373, "R^2"=w354, "MSE"=w374, "Best Fit Parameters"=w359) -> ("Array of Asymmetric Gaussian Fit Parameters"=w363:T8[])  [unwired: 6 in, 1 out]
          n157 = Index Array(array=w357) -> (element=w356:dbl)  [unwired: 1 in]
          n158 = Bundle(cluster=w362, "Asymmetric Gaussian Parameters"=w366, "Bridge Amplitude"=w364) -> (w371:T15)
          n159 = Bundle(cluster=w362, "Asymmetric Gaussian Parameters"=w363, "Bridge Amplitude"=w356) -> (w372:T15)
        }
        frame "Two T-Connected Asymmetric Gaussians" {
          w413 = T16 {"Asymmetric Gaussian Parameters"=[], "Bridge Amplitude"=0.0, "Bridge Slope"=0.0} ("Two T-Connected Asymmetric Gaussian Parameters")
          w411 = 0.0 ("MSE")
          n160 = Variant To Data(type=T5 {"Fix D-only Peak Location"=FALSE, "Peak Location"=0.0, "Fix D-only Peak FWHM"=FALSE, "Peak FWHM"=0.0} ("Fixed Parameters"), Variant=w443) -> (data=w442:T5)  [unwired: 1 in, 1 out]
          n161 = Unbundle By Name(w442) -> ("Fix D-only Peak FWHM"=w434:bool, "Peak FWHM"=w438:dbl, "Fix D-only Peak Location"=w436:bool, "Peak Location"=w439:dbl)
          n162 = case shown="True" w436 {
            tunnel: w441 -> [w465 w469]
            tunnel: [w465 w468] -> w440
            tunnel: w439 -> [_ w466]
            frame False {
            }
            frame True {
              n163 = Insert Into Array(array=w469, index=1 ("length"), new element=w466) -> (w468:dbl[])
            }
          }
          n164 = case shown="True" w434 {
            tunnel: w440 -> [w455 w460]
            tunnel: [w455 w464] -> w418
            tunnel: w438 -> [_ w462]
            frame False {
            }
            frame True {
              n165 = Index Array(array=w460, index=2) -> (element=w457:dbl)
              n166 = Absolute Value(x=w457) -> (abs(x)=w456:dbl)
              n167 = expression code="x/sqrt(2*ln(2))"(w462) -> (w461:dbl)
              n168 = Compound Arithmetic op=ADD(invert w456, w461) -> (w458:dbl)
              n169 = Insert Into Array(array=w460, index=3, new element=w458) -> (w464:dbl[])
            }
          }
          n170 = case shown="True" w436 {
            tunnel: w437 -> [w450 w454]
            tunnel: [w450 w453] -> w435
            frame False {
            }
            frame True {
              n171 = Insert Into Array(array=w454, index=1 ("length"), new element=0.0 ("new element/subarray")) -> (w453:dbl[])
            }
          }
          n172 = case shown="True" w434 {
            tunnel: w435 -> [w445 w449]
            tunnel: [w445 w448] -> w427
            frame False {
            }
            frame True {
              n173 = Insert Into Array(array=w449, index=3, new element=0.0 ("new element/subarray")) -> (w448:dbl[])
            }
          }
          n174 = Array Size(array=w427) -> (size(s)=w429:i32)
          n175 = Array Size(array=w418) -> (size(s)=w420:i32)
          n176 = expression code="x-2"(w429) -> (w428:i32)
          n177 = expression code="x-2"(w420) -> (w421:i32)
          n178 = Split 1D Array(array=w427, index=w428) -> (first subarray=w426:dbl[], second subarray=w424:dbl[])
          n179 = Split 1D Array(array=w418, index=w421) -> (first subarray=w419:dbl[], second subarray=w417:dbl[])
          n180 = call "Format Sum of Asymmetric Gaussians Fit Parameters.vi"("Step Size"=w411, "R^2"=w411, "MSE"=w411, "Best Fit Parameters"=w426) -> ("Array of Asymmetric Gaussian Fit Parameters"=w425:T8[])  [unwired: 6 in, 1 out]
          n181 = Index Array(array=w424) -> (element #1=w423:dbl, element #2=w415:dbl)  [unwired: 2 in]
          n182 = call "Format Sum of Asymmetric Gaussians Fit Parameters.vi"("Step Size"=w432, "R^2"=w412, "MSE"=w433, "Best Fit Parameters"=w419) -> ("Array of Asymmetric Gaussian Fit Parameters"=w422:T8[])  [unwired: 6 in, 1 out]
          n183 = Index Array(array=w417) -> (element #1=w416:dbl, element #2=w414:dbl)  [unwired: 2 in]
          n184 = Bundle By Name(cluster=w413, "Asymmetric Gaussian Parameters"=w425, "Bridge Amplitude"=w423, "Bridge Slope"=w415) -> (w430:T16)
          n185 = Bundle By Name(cluster=w413, "Asymmetric Gaussian Parameters"=w422, "Bridge Amplitude"=w416, "Bridge Slope"=w414) -> (w431:T16)
        }
        frame "Single Exponential" {
          w484 = T17 {"Amplitude"=0.0, "Time Constant"=0.0, "Mean"=0.0, "SDV"=0.0, "FWHM"=0.0, "Integral"=0.0, "MSE"=0.0, "R^2"=0.0} ("Single Exponential Fit Parameters")
          n186 = Index Array(array=w480) -> (element #1=w474:dbl, element #2=w478:dbl)  [unwired: 2 in]
          n187 = Index Array(array=w483) -> (element #1=w482:dbl, element #2=w481:dbl)  [unwired: 2 in]
          n188 = Multiply(x=w478, y=0.6931471805599453) -> (x*y=w477:dbl)
          n189 = Compound Arithmetic op=MULTIPLY(w474, w478, invert w475) -> (w473:dbl)
          n190 = Bundle By Name(cluster=w484, "Amplitude"=w482, "Time Constant"=w481) -> (w472:T17)
          n191 = Bundle By Name(cluster=w484, "Amplitude"=w474, "Time Constant"=w478, "Mean"=w478, "SDV"=w478, "FWHM"=w477, "Integral"=w473, "MSE"=w476, "R^2"=w470) -> (w471:T17)
        }
        frame "Two Exponentials" {
          w491 = T18 {"A1"=0.0, "tau1"=0.0, "A2"=0.0, "tau2"=0.0, "Mean"=0.0, "SDV"=0.0, "Integral"=0.0, "MSE"=0.0, "R^2"=0.0} ("Double Exponential Fit Parameters")
          n192 = Index Array(array=w497) -> (element #1=w489:dbl, element #2=w488:dbl, element #3=w487:dbl, element #4=w486:dbl)  [unwired: 4 in]
          n193 = formula code="float64 N;\nN = A1*t1+A2*t2;\nm = (A1*t1**2+A2*t2**2)/N;\ns = 2*sqrt(A1*t1*A2*t2)*abs(t2-t1)/N;\nI = (A1*t1 + A2*t2)/dt;"("t1"=w488, "A2"=w487, "t2"=w486, "dt"=w496, "A1"=w489) -> ("m"=w495:dbl, "s"=w494:dbl, "I"=w493:dbl)
          n194 = Index Array(array=w503) -> (element #1=w502:dbl, element #2=w501:dbl, element #3=w500:dbl, element #4=w499:dbl)  [unwired: 4 in]
          n195 = Bundle By Name(cluster=w491, "A1"=w489, "tau1"=w488, "A2"=w487, "tau2"=w486, "Mean"=w495, "SDV"=w494, "MSE"=w492, "Integral"=w493, "R^2"=w485) -> (w490:T18)
          n196 = Bundle By Name(cluster=w491, "A1"=w502, "tau1"=w501, "A2"=w500, "tau2"=w499) -> (w498:T18)
        }
        frame "2D Gaussian ACF" {
          w514 = T19 {"Amplitude"=0.0, "Diffusion Time"=0.0, "RMSE"=0.0, "R^2"=0.0} ("2D ACF Fit Parameters")
          n197 = Index Array(array=w509) -> (element #1=w508:dbl, element #2=w506:dbl)  [unwired: 2 in]
          n198 = Index Array(array=w512) -> (element #1=w505:dbl, element #2=w504:dbl)  [unwired: 2 in]
          n199 = Bundle By Name(cluster=w514, "Amplitude"=w508, "Diffusion Time"=w506) -> (w511:T19)
          n200 = Bundle By Name(cluster=w514, "Amplitude"=w505, "Diffusion Time"=w504, "RMSE"=w513, "R^2"=w507) -> (w510:T19)
        }
        frame "2D Gaussian + Blinking ACF" {
          w529 = T20 {"Amplitude"=0.0, "Diffusion Time"=0.0, "Blinking Fraction"=0.0, "Blinking Time Constant"=0.0, "RMSE"=0.0, "R^2"=0.0} ("2D Gaussian + Blinking ACF Fit Parameters")
          n201 = Index Array(array=w527) -> (element #1=w520:dbl, element #2=w519:dbl, element #3=w516:dbl, element #4=w515:dbl)  [unwired: 4 in]
          n202 = Index Array(array=w524) -> (element #1=w523:dbl, element #2=w521:dbl, element #3=w518:dbl, element #4=w517:dbl)  [unwired: 4 in]
          n203 = Bundle By Name(cluster=w529, "Amplitude"=w523, "Diffusion Time"=w521, "Blinking Fraction"=w518, "Blinking Time Constant"=w517) -> (w526:T20)
          n204 = Bundle By Name(cluster=w529, "Amplitude"=w520, "Diffusion Time"=w519, "Blinking Fraction"=w516, "Blinking Time Constant"=w515, "RMSE"=w528, "R^2"=w522) -> (w525:T20)
        }
        frame "2D Gaussian + Flow ACF" {
          w542 = T21 {"Amplitude"=0.0, "Diffusion Time"=0.0, "Translation Time"=0.0, "RMSE"=0.0, "R^2"=0.0} ("2D Gaussian + Blinking ACF Fit Parameters")
          n205 = Index Array(array=w540) -> (element #1=w533:dbl, element #2=w532:dbl, element #3=w530:dbl)  [unwired: 3 in]
          n206 = Index Array(array=w537) -> (element #1=w536:dbl, element #2=w534:dbl, element #3=w531:dbl)  [unwired: 3 in]
          n207 = Bundle By Name(cluster=w542, "Amplitude"=w536, "Diffusion Time"=w534, "Translation Time"=w531) -> (w539:T21)
          n208 = Bundle By Name(cluster=w542, "Amplitude"=w533, "Diffusion Time"=w532, "Translation Time"=w530, "RMSE"=w541, "R^2"=w535) -> (w538:T21)
        }
        frame "3D Gaussian ACF" {
          w547 = T22 {"Amplitude"=0.0, "Diffusion Time"=0.0, "Aspect Ratio"=0.0, "RMSE"=0.0, "R^2"=0.0} ("3D ACF Fit Parameters")
          n209 = Index Array(array=w552) -> (element #1=w545:dbl, element #2=w550:dbl, element #3=w546:dbl)  [unwired: 3 in]
          n210 = Index Array(array=w555) -> (element #1=w549:dbl, element #2=w548:dbl, element #3=w544:dbl)  [unwired: 3 in]
          n211 = Absolute Value(x=w544) -> (abs(x)=w543:dbl)
          n212 = Bundle By Name(cluster=w547, "Amplitude"=w545, "Diffusion Time"=w550, "Aspect Ratio"=w546) -> (w554:T22)
          n213 = Bundle By Name(cluster=w547, "Amplitude"=w549, "Diffusion Time"=w548, "Aspect Ratio"=w543, "RMSE"=w556, "R^2"=w551) -> (w553:T22)
        }
        frame "3D Gaussian + Blinking ACF" {
          w563 = T23 {"Amplitude"=0.0, "Diffusion Time"=0.0, "Aspect Ratio"=0.0, "Blinking Fraction"=0.0, "Blinking Time Constant"=0.0, "RMSE"=0.0, "R^2"=0.0} ("2D Gaussian + Blinking ACF Fit Parameters")
          n214 = Index Array(array=w572) -> (element #1=w565:dbl, element #2=w564:dbl, element #3=w557:dbl, element #4=w558:dbl, element #5=w559:dbl)  [unwired: 5 in]
          n215 = Index Array(array=w569) -> (element #1=w568:dbl, element #2=w566:dbl, element #3=w560:dbl, element #4=w561:dbl, element #5=w562:dbl)  [unwired: 5 in]
          n216 = Bundle By Name(cluster=w563, "Amplitude"=w565, "Diffusion Time"=w564, "Aspect Ratio"=w557, "Blinking Fraction"=w558, "Blinking Time Constant"=w559, "RMSE"=w573, "R^2"=w567) -> (w570:T23)
          n217 = Bundle By Name(cluster=w563, "Amplitude"=w568, "Diffusion Time"=w566, "Aspect Ratio"=w560, "Blinking Fraction"=w561, "Blinking Time Constant"=w562) -> (w571:T23)
        }
        frame "2D Gaussian ACF & 2D Gaussian + Flow ACF" {
          w576 = T24 {"Amplitude 1"=0.0, "Diffusion Time"=0.0, "Amplitude 2"=0.0, "Translation Time"=0.0, "RMSE"=0.0, "R^2"=0.0} ("2D Gaussian ACF & ACF + Flow Fit Parameters")
          n218 = Index Array(array=w584) -> (element #1=w583:dbl, element #2=w581:dbl, element #3=w575:dbl, element #4=w578:dbl)  [unwired: 4 in]
          n219 = Index Array(array=w587) -> (element #1=w580:dbl, element #2=w579:dbl, element #3=w574:dbl, element #4=w577:dbl)  [unwired: 4 in]
          n220 = Bundle By Name(cluster=w576, "Amplitude 1"=w583, "Diffusion Time"=w581, "Amplitude 2"=w575, "Translation Time"=w578) -> (w586:T24)
          n221 = Bundle By Name(cluster=w576, "Amplitude 1"=w580, "Diffusion Time"=w579, "Amplitude 2"=w574, "Translation Time"=w577, "RMSE"=w588, "R^2"=w582) -> (w585:T24)
        }
      }
    }
    frame Error {
    }
  }
  "Fit Parameters Cluster" <- w8
  "Fit Parameters Uncertainties Cluster" <- w9
  "Error Out" <- w2
